vi "Update Basic Components.vi"(8 "error in (no error)":errorcluster, 11 "HistorianCharting in":refnum<class "HistorianCharting.lvclass">) -> (0 "error out":errorcluster, 3 "HistorianCharting out":refnum<class "HistorianCharting.lvclass">)   [LabVIEW 2020, in "VolatusGUIElements.lvlib" / "HistorianCharting.lvclass"]
uses:
  HistorianCharting.lvclass
  HistorianCharting.lvclass/HistorianCharting.ctl
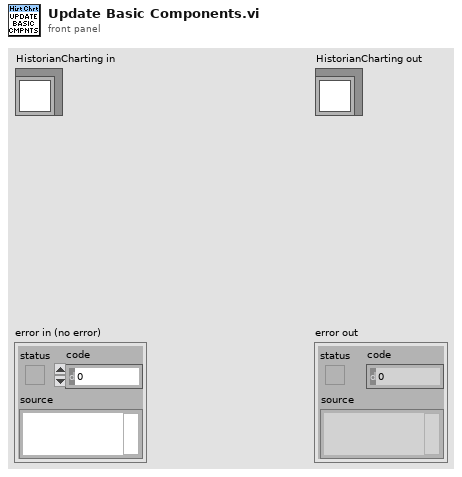
[diagram p1: front panel]
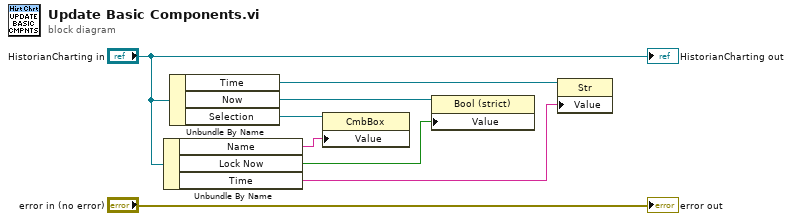
[diagram p0: block diagram]
diagram:
  n1 = Unbundle By Name("HistorianCharting in") -> ("Name"=w5:string, "Lock Now"=w3:bool, "Time"=w1:string)
  n2 = Unbundle By Name("HistorianCharting in") -> ("Time"=w2:refnum<vi>, "Now"=w4:refnum<vi>, "Selection"=w6:refnum<vi>)
  n3 = property class="CmbBox"(reference=w6, "Value"=w5) -> ()  [unwired: 1 in, 2 out]
  n4 = property class="Bool (strict)"(reference=w4, "Value"=w3) -> ()  [unwired: 1 in, 2 out]
  n5 = property class="Str"(reference=w2, "Value"=w1) -> ()  [unwired: 1 in, 2 out]
  "error out" <- "error in (no error)"
  "HistorianCharting out" <- "HistorianCharting in"
